vi "control.vi"() -> ()   [LabVIEW 2018]
panel:
  out "PWM":dbl
  in  "Angle":dbl
  in  "Encoder":dbl
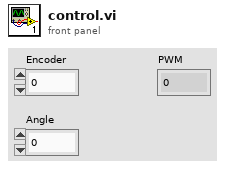
[diagram p1: front panel]
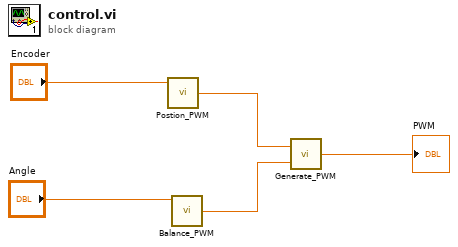
[diagram p0: block diagram]
diagram:
  n1 = call "Postion_PWM.vi"("Encoder"="Encoder") -> ("Postion_PWM"=w3:dbl)  [unwired: 2 in]
  n2 = call "Balance_PWM.vi"("Angle"="Angle") -> ("Balance_PWM"=w2:dbl)  [unwired: 3 in]
  n3 = call "Generate_PWM.vi"("Balance_PWM"=w2, "Position_PWM"=w3) -> ("PWM"=→"PWM":dbl)
